vi "探头滤波次数.vi"(7 "校准参数":u16(ring) caption="校准参数：" items=["pH", "DO", "浊度", "电导率", "叶绿素a", "藻密度", "ORP", "DO2", "氯化物"], 8 "error in (no error)":errorcluster caption="错误输入（无错误）", 11 "滤波次数":u32) -> (0 "error out":errorcluster caption="错误输出")   [LabVIEW 2022 SP3, in "斯坦道多参数.lvlib"]
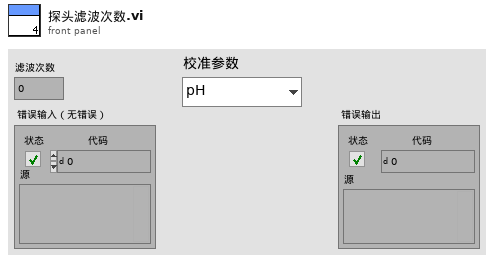
[diagram p1: front panel]
types:
  T1 = typedef "斯坦道多参数.lvlib/探头类型.ctl" = enum16{"禹山", "国弘", "纳清", "STD"}
  T2 = enum16{"NULL", "pH", "Cond", "DO", "Turb", "ORP"}
  T3 = enum16{"NULL", "pH", "Cond", "DO", "Turb", "ORP", "6", "7", "8", "9", "氯化物"}
  T4 = cluster{"pH":u32, "DO":u32, "Cond":u32, "Turb":u32, "叶绿素a":u32, "藻密度":u32, "ORP":u32, "COD":u32, "氯化物":u32, "氨氮":u32, "水中油":u32, "悬浮物":u32, "余氯":u32}
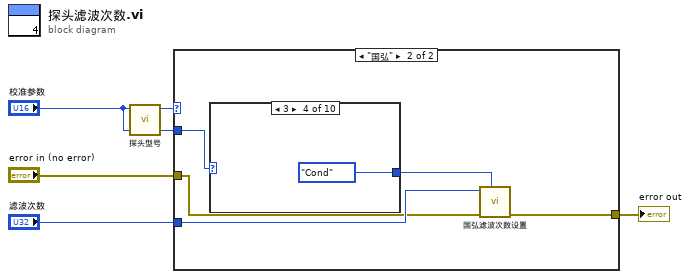
[diagram p0: block diagram]
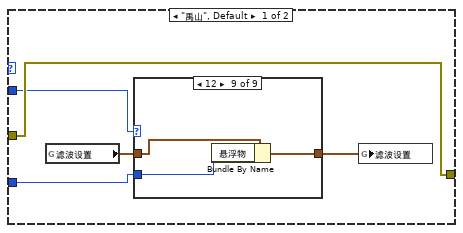
[diagram p2: hidden frame]
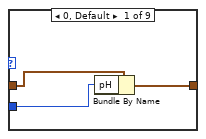
[diagram p3: hidden frame]
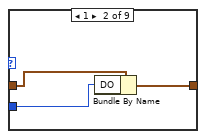
[diagram p4: hidden frame]
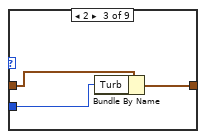
[diagram p5: hidden frame]
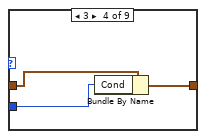
[diagram p6: hidden frame]
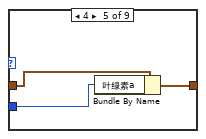
[diagram p7: hidden frame]
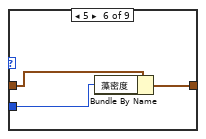
[diagram p8: hidden frame]
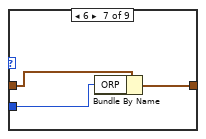
[diagram p9: hidden frame]
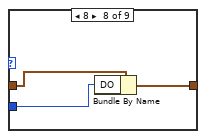
[diagram p10: hidden frame]
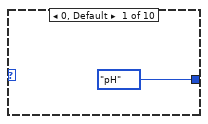
[diagram p11: hidden frame]
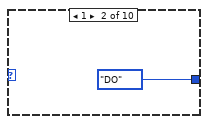
[diagram p12: hidden frame]
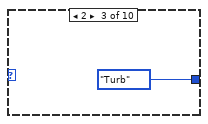
[diagram p13: hidden frame]
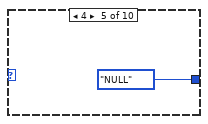
[diagram p14: hidden frame]
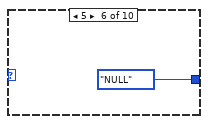
[diagram p15: hidden frame]
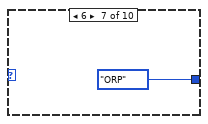
[diagram p16: hidden frame]
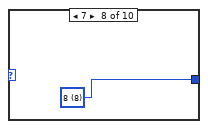
[diagram p17: hidden frame]
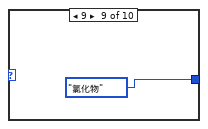
[diagram p18: hidden frame]
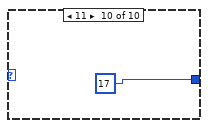
[diagram p19: hidden frame]
diagram:
  n1 = call "探头型号.vi"("校准参数"="校准参数") -> ("探头型号"=w5:T1)  [unwired: 8 in, 2 out]
  n2 = case shown="\"国弘\"" w5 {
    tunnel: "校准参数" -> [w7 w42]
    tunnel: "error in (no error)" -> [w10 w39]
    tunnel: [w10 w38] -> w2
    tunnel: "滤波次数" -> [w6 w40]
    frame "禹山", Default {
      n3 = global read "断电保存变量.vi" "滤波设置"() -> (w9:T4)
      n4 = case shown="12" w7 {
        tunnel: w6 -> [w11 w15 w17 w20 w23 w26 w29 w32 w35]
        tunnel: w9 -> [w13 w16 w19 w22 w24 w27 w31 w33 w36]
        tunnel: [w12 w14 w18 w21 w25 w28 w30 w34 w37] -> w8
        frame 0, Default {
          n5 = Bundle By Name(cluster=w13, "pH"=w11) -> (w12:T4)
        }
        frame 1 {
          n6 = Bundle By Name(cluster=w16, "DO"=w15) -> (w14:T4)
        }
        frame 2 {
          n7 = Bundle By Name(cluster=w19, "Turb"=w17) -> (w18:T4)
        }
        frame 3 {
          n8 = Bundle By Name(cluster=w22, "Cond"=w20) -> (w21:T4)
        }
        frame 4 {
          n9 = Bundle By Name(cluster=w24, "叶绿素a"=w23) -> (w25:T4)
        }
        frame 5 {
          n10 = Bundle By Name(cluster=w27, "藻密度"=w26) -> (w28:T4)
        }
        frame 6 {
          n11 = Bundle By Name(cluster=w31, "ORP"=w29) -> (w30:T4)
        }
        frame 8 {
          n12 = Bundle By Name(cluster=w33, "DO"=w32) -> (w34:T4)
        }
        frame 12 {
          n13 = Bundle By Name(cluster=w36, "悬浮物"=w35) -> (w37:T4)
        }
      }
      n14 = global write "断电保存变量.vi" "滤波设置"(w8) -> ()
    }
    frame "国弘" {
      n15 = case shown="3" w42 {
        tunnel: [T2."pH" ("探头") T2."DO" ("探头") T2."Turb" ("探头") T2."Cond" ("探头") T2."NULL" ("探头") T2."NULL" ("探头") T2."ORP" ("探头") w50 T3."氯化物" ("探头") 17] -> w41
        frame 0, Default {
        }
        frame 1 {
        }
        frame 2 {
        }
        frame 3 {
        }
        frame 4 {
        }
        frame 5 {
        }
        frame 6 {
        }
        frame 7 {
          w50 = u16 8 items=["NULL", "pH", "Cond", "DO", "Turb", "ORP", "6", "7", "8", "9", "氯化物"] ("探头")
        }
        frame 9 {
        }
        frame 11 {
        }
      }
      n16 = call "国弘滤波次数设置.vi"("探头"=w41, "error in (no error)"=w39, "滤波次数"=w40) -> ("error out"=w38:errorcluster)  [unwired: 7 in, 1 out]
    }
  }
  "error out" <- w2
